vi "mod_Continuous BB-PAM generation.vi"(0 "Bit stream":T1(tab), 1 "Symbol Rate, Hz":dbl=1.0 format="%.2f", 2 "PAM system parameters":T2={"samples per symbol (16)"=16, "symbol map"=[]} {"symbol map" format="%.3f"}, 5 "PN Sequence Order":i32=9, 9 "user base bit pattern":i8[](array[numeric]), 11 "error in (no error)":errorcluster, 12 "filter parameters":T3={"Alpha"=0.5, "Filter Length"=6, "TX Filter"=enum."Root Raised Cos"} {"Alpha" format="%.2f"}, 13 "Path":path) -> (4 "output complex waveform":T4 {"Y" format="%.3f"; "dt" format="%^.2e"; "t0" format="%.4f"}, 15 "error out":errorcluster)   [LabVIEW 2020, in "niDMT.lvlib"]
uses:
  <vilib>/addons/Modulation/niDMT.lvlib
  <vilib>/addons/Modulation/Analog/controls/Complex Data Waveform.ctl
  <vilib>/addons/Modulation/Digital/Support/Controls/PAM system parameters.ctl
  <vilib>/addons/Modulation/Digital/General/MT Generate Bits (Galois, PN Order).vi
  <vilib>/addons/Modulation/Digital/Support/Common/Validators/mod_Generate Bits Validate.vi
  <vilib>/addons/Modulation/Analog/support/mod_Set Error Source.vi
  <vilib>/addons/Modulation/Digital/General/subVIs/mod_Generate Bits PN Sequence.vi
  <vilib>/addons/Modulation/Digital/General/MT Generate Bits (User Defined).vi
  <vilib>/Utility/file.llb/Read From Spreadsheet File (DBL).vi
  <vilib>/addons/Modulation/Digital/Support/Common/Validators/mod_Generate Filter Coefficients Validate.vi
  <vilib>/addons/Modulation/Digital/General/subVIs/mod_Generate Filter Coefficients.vi
  <vilib>/addons/Modulation/niAMT.lvlib
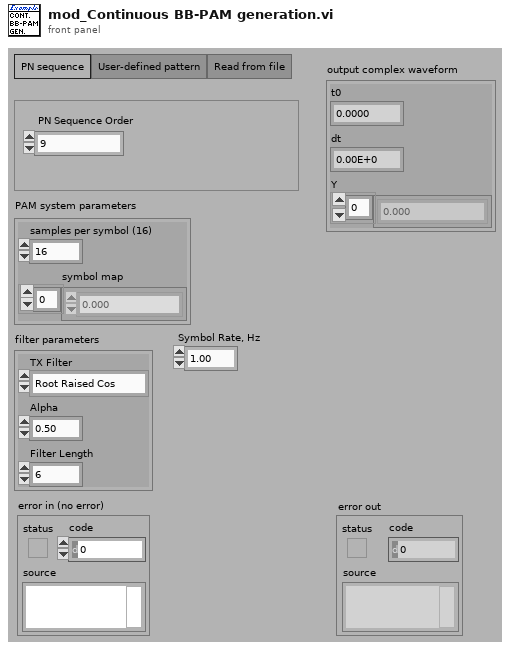
[diagram p1: front panel]
types:
  T1 = enum32{"PN sequence", "User-defined pattern", "Read from file"}
  T2 = typedef "niDMT.lvlib/PAM system parameters.ctl" = cluster{"samples per symbol (16)":i32, "symbol map":cdb[]}
  T3 = cluster{"Alpha":dbl, "Filter Length":i32, "TX Filter":enum16{"none", "Raised Cosine", "Root Raised Cos", "Gaussian"}}
  T4 = typedef "niAMT.lvlib/Complex Data Waveform.ctl" = cluster{"t0":dbl, "dt":dbl, "Y":cdb[]}
  T5 = enum16{"none", "Raised Cosine", "Root Raised Cos", "Gaussian"}
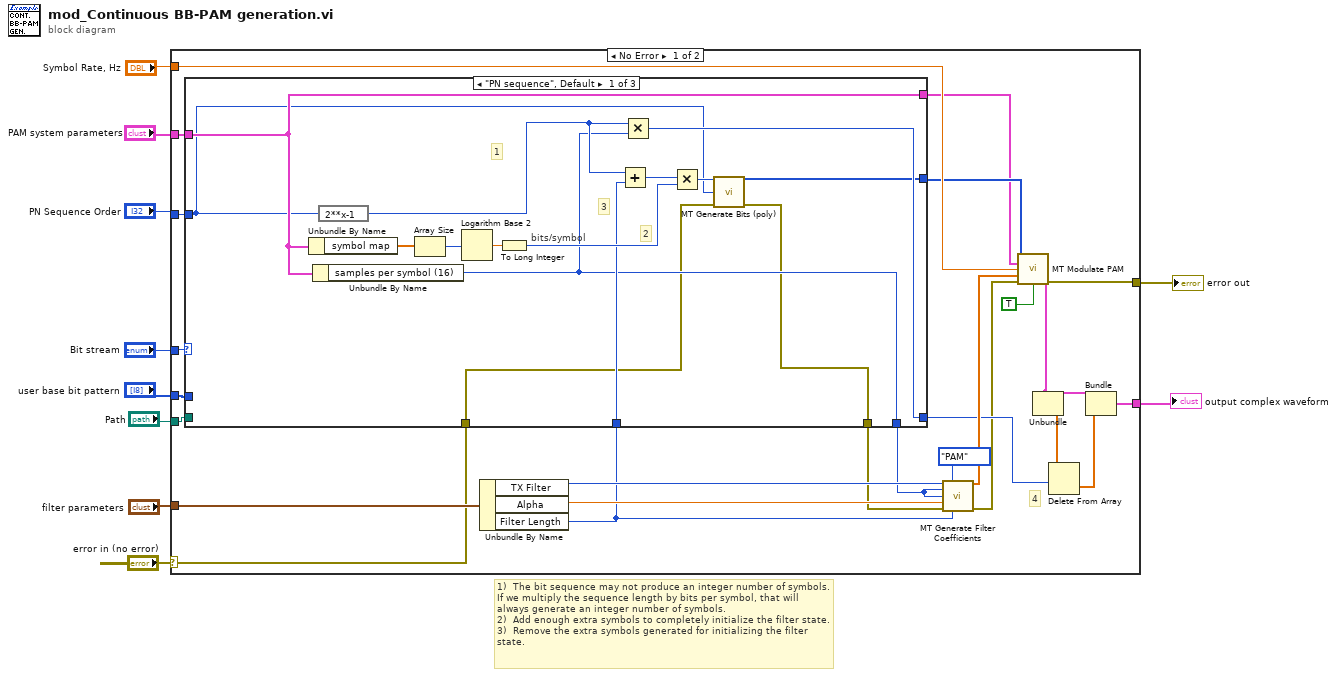
[diagram p0: block diagram]
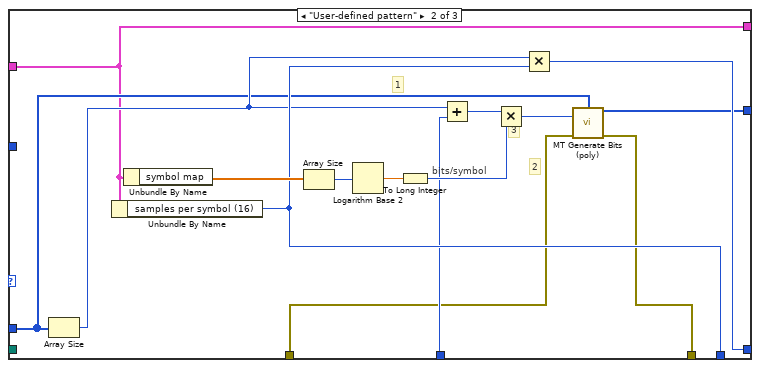
[diagram p2: hidden frame]
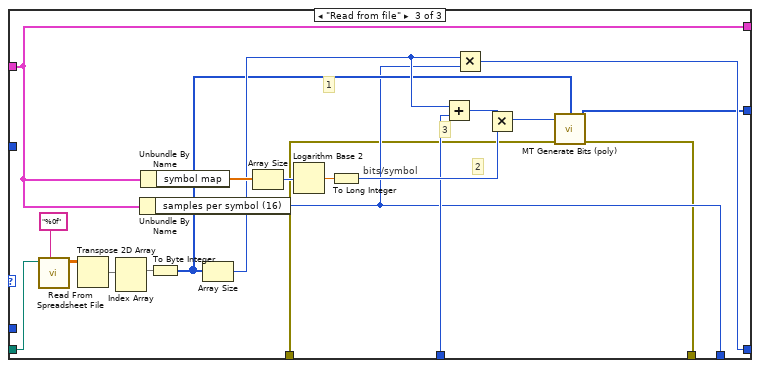
[diagram p3: hidden frame]
diagram:
  # "1)  The bit sequence may not produce an integer number of symbols.  If we multiply the sequence length by bits per symbol, that will always generate an integer number of symbols. \n2)  Add enough extra symbols to completely initialize the filter state.\n3)  Remove the extra symbols generated for initializing the filter state."
  n1 = case shown="No Error" "error in (no error)" {
    selector: "error in (no error)" -> [w13 w86]
    tunnel: [w35 _] -> w10
    tunnel: [w34 w86] -> w9
    tunnel: "Symbol Rate, Hz" -> [w31 _]
    tunnel: "PN Sequence Order" -> [w20 _]
    tunnel: "user base bit pattern" -> [w30 _]
    tunnel: "Bit stream" -> [w22 _]
    tunnel: "filter parameters" -> [w29 _]
    tunnel: "PAM system parameters" -> [w19 _]
    tunnel: "Path" -> [w21 _]
    frame No Error {
      # "4"
      n2 = Unbundle By Name(w29) -> ("TX Filter"=w32:T5, "Alpha"=w33:dbl, "Filter Length"=w11:i32)
      n3 = case shown="\"PN sequence\", Default" w22 {
        tunnel: w30 -> [_ w55 _]
        tunnel: w20 -> [w38 _ _]
        tunnel: w21 -> [_ _ w82]
        tunnel: w19 -> [w41 w53 w69]
        tunnel: [w42 w59 w71] -> w18
        tunnel: [w40 w58 w70] -> w17
        tunnel: w11 -> [w43 w56 w72]
        tunnel: [w39 w54 w68] -> w16
        tunnel: [w41 w53 w69] -> w15
        tunnel: w13 -> [w37 w52 w67]
        tunnel: [w36 w51 w66] -> w12
        frame "PN sequence", Default {
          # "2"
          # "1"
          # "3"
          # "bits/symbol"
          n4 = Unbundle By Name(w41) -> ("symbol map"=w45:cdb[])
          n5 = Unbundle By Name(w41) -> ("samples per symbol (16)"=w42:i32)
          n6 = expression code="2**x-1"(w38) -> (w44:i32)
          n7 = Array Size(array=w45) -> (size(s)=w46:i32)
          n8 = Logarithm Base 2(1:w46) -> (0:w47:dbl)
          n9 = To Long Integer(number=w47) -> (32bit integer=w48:i32)
          n10 = Add(x=w44, y=w43) -> (x+y=w49:i32)
          n11 = Multiply(x=w44, y=w42) -> (x*y=w40:i32)
          n12 = Multiply(x=w49, y=w48) -> (x*y=w50:i32)
          n13 = call-poly <vilib>:"MT Generate Bits (poly).vi"("total bits (128)"=w50, "PN sequence order (9)"=w38, "error in (no error)"=w37) -> ("output bit stream"=w39:i8[], "error out"=w36:errorcluster)  [unwired: 2 in, 9 out]
        }
        frame "User-defined pattern" {
          # "2"
          # "1"
          # "3"
          # "bits/symbol"
          n14 = Array Size(array=w55) -> (size(s)=w57:i32)
          n15 = Unbundle By Name(w53) -> ("samples per symbol (16)"=w59:i32)
          n16 = Unbundle By Name(w53) -> ("symbol map"=w60:cdb[])
          n17 = Array Size(array=w60) -> (size(s)=w61:i32)
          n18 = Logarithm Base 2(1:w61) -> (0:w62:dbl)
          n19 = To Long Integer(number=w62) -> (32bit integer=w63:i32)
          n20 = Add(x=w57, y=w56) -> (x+y=w64:i32)
          n21 = Multiply(x=w64, y=w63) -> (x*y=w65:i32)
          n22 = Multiply(x=w57, y=w59) -> (x*y=w58:i32)
          n23 = call-poly <vilib>:"MT Generate Bits (poly).vi"("total bits (128)"=w65, "user base bit pattern"=w55, "error in (no error)"=w52) -> ("output bit stream"=w54:i8[], "error out"=w51:errorcluster)  [unwired: 2 in, 9 out]
        }
        frame "Read from file" {
          # "2"
          # "1"
          # "3"
          # "bits/symbol"
          n24 = call-poly <vilib>:"Read From Spreadsheet File.vi"("format (%.3f)"="%0f", "file path (dialog if empty)"=w82) -> ("all rows"=w83:dbl[][])  [unwired: 2 in, 7 out]
          n25 = Transpose 2D Array(2D array=w83) -> (transposed array=w84:dbl[][])
          n26 = Index Array(array=w84) -> (element=w85:dbl[])  [unwired: 2 in]
          n27 = Unbundle By Name(w69) -> ("samples per symbol (16)"=w71:i32)
          n28 = Unbundle By Name(w69) -> ("symbol map"=w75:cdb[])
          n29 = To Byte Integer(number=w85) -> (8bit integer=w73:i8[])
          n30 = Array Size(array=w73) -> (size(s)=w74:i32)
          n31 = Array Size(array=w75) -> (size(s)=w76:i32)
          n32 = Logarithm Base 2(1:w76) -> (0:w77:dbl)
          n33 = To Long Integer(number=w77) -> (32bit integer=w78:i32)
          n34 = Add(x=w74, y=w72) -> (x+y=w79:i32)
          n35 = Multiply(x=w74, y=w71) -> (x*y=w70:i32)
          n36 = Multiply(x=w79, y=w78) -> (x*y=w80:i32)
          n37 = call-poly <vilib>:"MT Generate Bits (poly).vi"("total bits (128)"=w80, "user base bit pattern"=w73, "error in (no error)"=w67) -> ("output bit stream"=w68:i8[], "error out"=w66:errorcluster)  [unwired: 2 in, 9 out]
        }
      }
      n38 = call <vilib>:"MT Generate Filter Coefficients.vi"("pulse shaping filter (none)"=w32, "modulation type"=enum16{"FSK", "PSK", "QAM", "MSK", "PAM", "ASK"}."PAM", "pulse shaping samples per symbol (16)"=w18, "matched samples per symbol (16)"=w18, "filter parameter"=w33, "error in (no error)"=w12, "filter length (symbols)"=w11) -> ("pulse shaping filter coefficients"=w26:dbl[], "error out"=w14:errorcluster)  [unwired: 7 out]
      n39 = call <vilib>:"MT Modulate PAM.vi"("input bit stream"=w16, "PAM system parameters"=w15, "symbol rate (Hz)"=w31, "pulse shaping filter coefficients"=w26, "error in (no error)"=w14, "reset? (T)"=TRUE ("Reset (T)")) -> ("output complex waveform"=w28:T4, "error out"=w34:errorcluster)  [unwired: 1 in, 7 out]
      n40 = Unbundle(w28) -> ("Y"=w24:cdb[])  [unwired: 2 out]
      n41 = Delete From Array(array=w24, length=w17) -> (deleted portion=w25:cdb[])  [unwired: 1 in, 1 out]
      n42 = Bundle(cluster=w28, "Y"=w25) -> (w35:T4)  [unwired: 2 out]
    }
    frame Error {
    }
  }
  "error out" <- w9
  "output complex waveform" <- w10
